vi "fp5.vi"   [LabVIEW 2016]
uses:
  <vilib>/NXT/Block Support/NXT_OutputPort.ctl
  <vilib>/NXT/Block Support/NXT_InputPort.ctl
  <vilib>/NXT/NXTIO Xnodes/NXTIONodeSubVIs/LEGOResetMotors.vi
  <vilib>/NXT/Dual Mode Library/Sensors/Touch_Released.vi
  <vilib>/NXT/Dual Mode Library/Sensors/EV3_Color_Reflect.vi
  <vilib>/NXT/NXTIO Xnodes/NXTIONodeSubVIs/NXTMoveMotors.vi
  <vilib>/NXT/NXTIO Xnodes/NXTIONodeSubVIs/NXTMotorRunDistance.vi
  <vilib>/NXT/NXTIO Xnodes/NXTIONodeSubVIs/NXTStopMotors.vi
  <vilib>/NXT/Dual Mode Library/Sound/PlayF.vi
  <vilib>/NXT/Dual Mode Library/Sound/PlayG.vi
  <vilib>/NXT/Subs/LVHSConnector.ctl
  <vilib>/NXT/NXTIO Xnodes/AddressXNode/NXTIOAddress.xnode
  <vilib>/NXT/NXTIO Xnodes/NXTIOXNode/NXTIO.xnode
  <vilib>/NXT/LegoClasses/BrickReference/BrickReference.lvclass
types:
  T1 = typedef "NXT_OutputPort.ctl" = u8
  T2 = typedef "NXT_InputPort.ctl" = u32
  T3 = typedef "LVHSConnector.ctl" = refnum<class "BrickReference.lvclass">
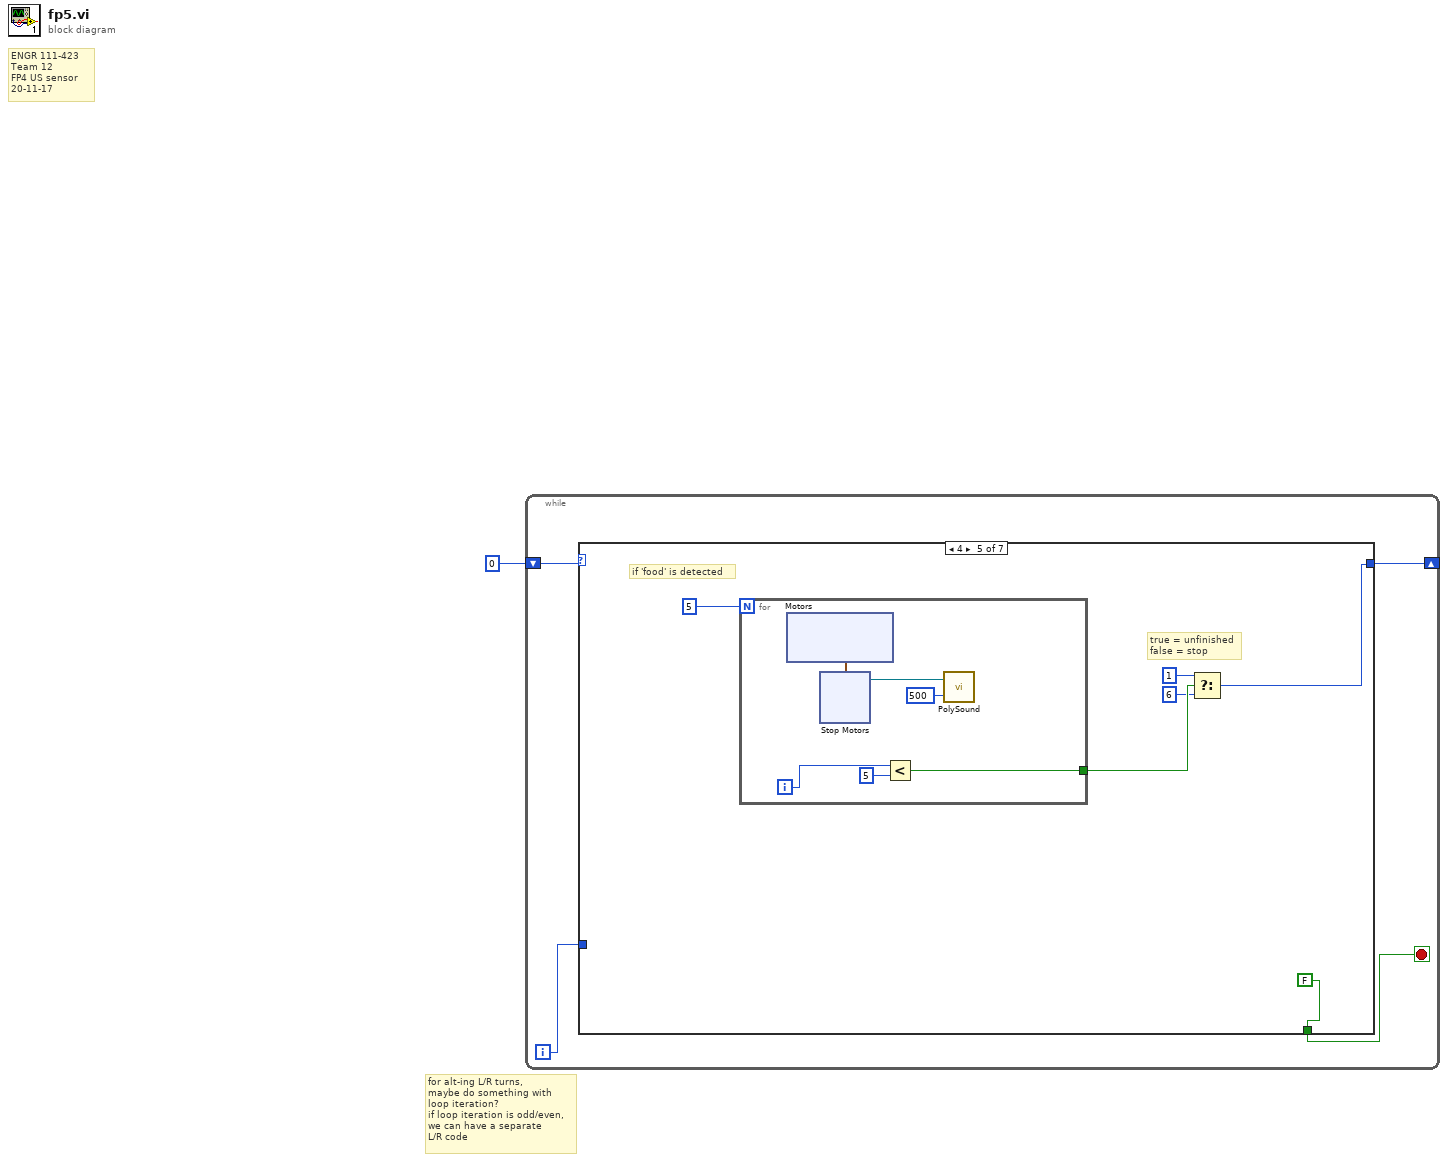
[diagram p0: block diagram]
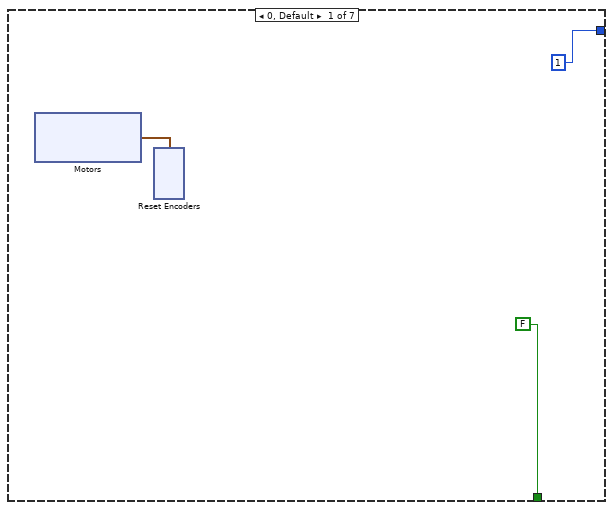
[diagram p2: hidden frame]
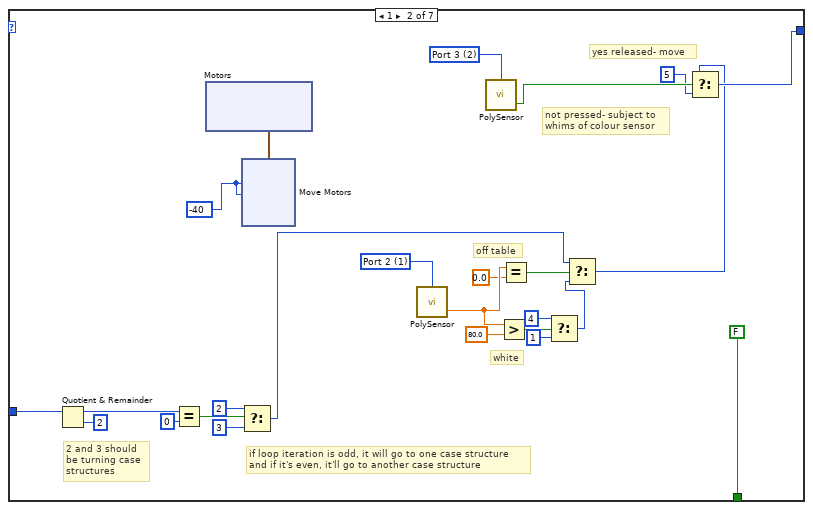
[diagram p3: hidden frame]
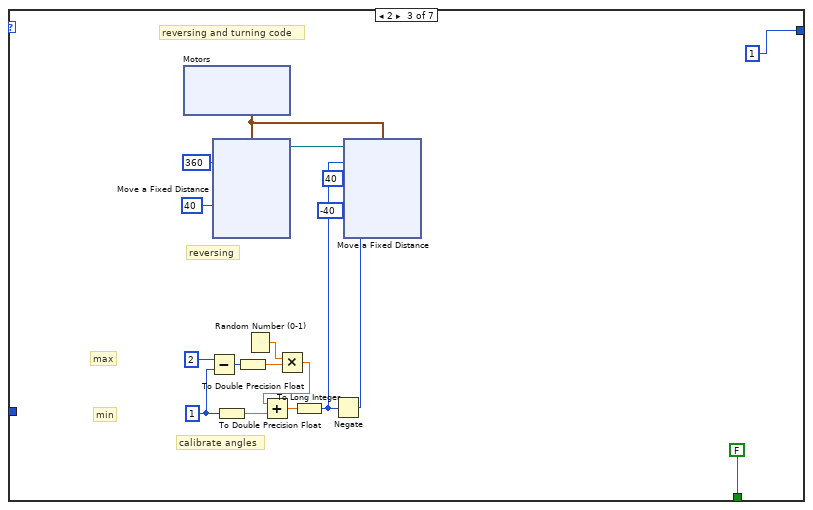
[diagram p4: hidden frame]
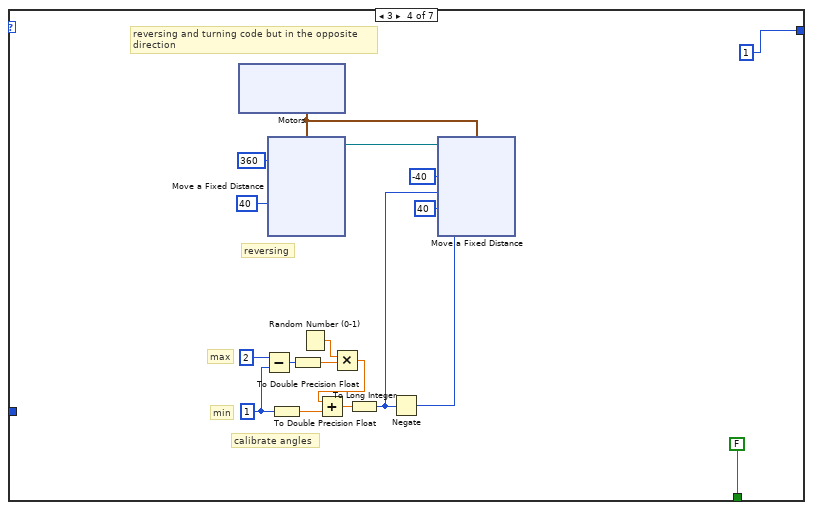
[diagram p5: hidden frame]
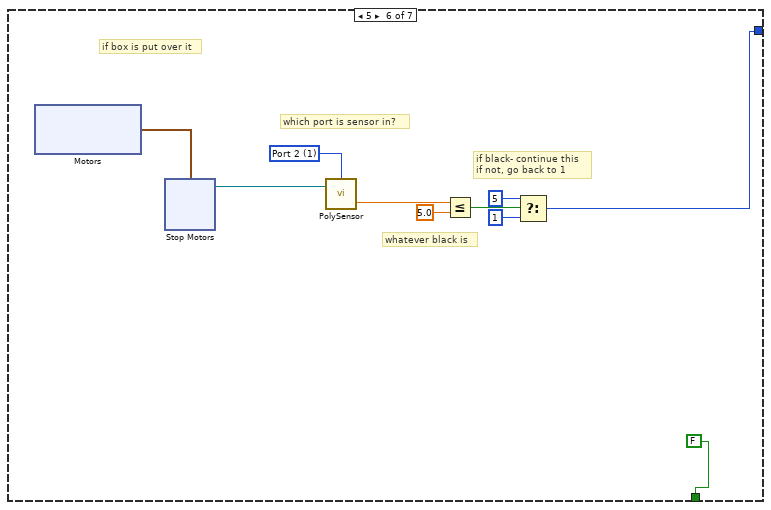
[diagram p6: hidden frame]
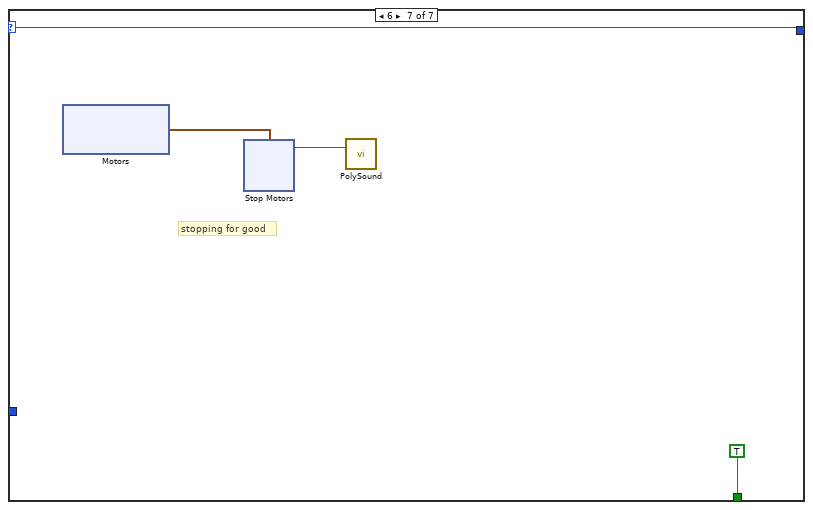
[diagram p7: hidden frame]
diagram:
  # "for alt-ing L/R turns,\nmaybe do something with\nloop iteration?\nif loop iteration is odd/even,\nwe can have a separate\nL/R code"
  # "ENGR 111-423\nTeam 12\nFP4 US sensor\n20-11-17"
  n1 = while {
    shift-right: [w3] -> _
    shift-left: 0 -> [w5]
    i -> [w2]
    stop <- w4 stop-if-true
    n2 = case shown="4" w5 {
      selector: w5 -> [_ _ _ _ _ _ w170]
      tunnel: [FALSE FALSE FALSE FALSE FALSE FALSE TRUE] -> w4
      tunnel: [1 w20 1 1 w135 w153 w170] -> w3
      tunnel: w2 -> [_ w33 _ _ _ _ _]
      frame 0, Default {
        n3 = xnode "Motors"() -> ("Motor"=w6:cluster{"Port":T1, "Port":T1})
        n4 = xnode "Reset Encoders"("Motors"=w6) -> ()  [unwired: 1 in, 1 out]
      }
      frame 1 {
        w21 = T2 1 items=["Port 1", "Port 2", "Port 3", "Port 4"] ("Port (Port 1)")
        w36 = T2 2 items=["Port 1", "Port 2", "Port 3", "Port 4"] ("Port (Port 1)")
        w37 = -40 ("Distance 1")
        # "white"
        # "off table"
        # "2 and 3 should\nbe turning case\nstructures"
        # "if loop iteration is odd, it will go to one case structure\nand if it's even, it'll go to another case structure"
        # "not pressed- subject to\nwhims of colour sensor"
        # "yes released- move"
        n5 = Quotient & Remainder(x=w33, y=2) -> (x-y*floor(x/y)=w31:i32)  [unwired: 1 out]
        n6 = Equal?(x=w31, y=0) -> (x = y?=w29:bool)
        n7 = xnode "Motors"() -> ("Motor"=w38:cluster{"Port":T1, "Port":T1})
        n8 = xnode "Move Motors"("Power/Speed 2"=w37, "Power/Speed 1"=w37, "Motors"=w38) -> ()  [unwired: 1 in, 1 out]
        n9 = Select(t=i16 2, s=w29, f=i16 3) -> (s? t:f=w18:i16)
        n10 = call-poly <vilib>:"PolySensor.vi"("Port (Port 1)"=w21) -> ("Scaled Value"=w22:sgl)  [unwired: 2 in, 1 out]
        n11 = call-poly <vilib>:"PolySensor.vi"("Port (Port 1)"=w36) -> ("Yes / No"=w35:bool)  [unwired: 2 in, 1 out]
        n12 = Greater?(x=w22, y=sgl 80.0) -> (0:w26:bool)
        n13 = Equal?(x=w22, y=sgl 0.0) -> (x = y?=w24:bool)
        n14 = Select(t=i16 4, s=w26, f=i16 1) -> (s? t:f=w17:i16)
        n15 = Select(t=w18, s=w24, f=w17) -> (s? t:f=w14:i16)
        n16 = Select(t=w14, s=w35, f=i16 5 ("t")) -> (s? t:f=w20:i16)
      }
      frame 2 {
        w58 = 1
        w64 = i8 40 ("Speed 2")
        w65 = 360 ("Distance 1")
        # "calibrate angles"
        # "min"
        # "max"
        # "reversing"
        # "reversing and turning code"
        n17 = xnode "Motors"() -> ("Motor"=w55:cluster{"Port":T1, "Port":T1})
        n18 = Subtract(x=2, y=w58) -> (x-y=w57:i32)
        n19 = xnode "Move a Fixed Distance"("Speed 2"=w64, "Speed 1"=w64, "Distance 2"=w65, "Distance 1"=w65, "Motors"=w55) -> ("NXT/EV3"=w54:T3)  [unwired: 1 in]
        n20 = To Double Precision Float(number=w58) -> (double precision float=w59:dbl)
        n21 = To Double Precision Float(number=w57) -> (double precision float=w60:dbl)
        n22 = Random Number (0-1)() -> (number: 0 to 1=w61:dbl)
        n23 = Multiply(x=w61, y=w60) -> (x*y=w63:dbl)
        n24 = Add(x=w63, y=w59) -> (x+y=w62:dbl)
        n25 = To Long Integer(number=w62) -> (32bit integer=w53:i32)
        n26 = Negate(x=w53) -> (-x=w52:i32)
        n27 = xnode "Move a Fixed Distance"("Speed 2"=i8 -40, "Speed 1"=i8 40, "Distance 2"=w52, "Distance 1"=w53, "Motors"=w55, "NXT/EV3"=w54) -> ()  [unwired: 1 out]
      }
      frame 3 {
        w104 = 1
        w98 = i8 40 ("Speed 2")
        w97 = 360 ("Distance 1")
        # "reversing and turning code but in the opposite\ndirection"
        # "calibrate angles"
        # "min"
        # "max"
        # "reversing"
        n28 = xnode "Motors"() -> ("Motor"=w107:cluster{"Port":T1, "Port":T1})
        n29 = Subtract(x=2, y=w104) -> (x-y=w105:i32)
        n30 = xnode "Move a Fixed Distance"("Speed 2"=w98, "Speed 1"=w98, "Distance 2"=w97, "Distance 1"=w97, "Motors"=w107) -> ("NXT/EV3"=w108:T3)  [unwired: 1 in]
        n31 = To Double Precision Float(number=w104) -> (double precision float=w103:dbl)
        n32 = To Double Precision Float(number=w105) -> (double precision float=w102:dbl)
        n33 = Random Number (0-1)() -> (number: 0 to 1=w101:dbl)
        n34 = Multiply(x=w101, y=w102) -> (x*y=w99:dbl)
        n35 = Add(x=w99, y=w103) -> (x+y=w100:dbl)
        n36 = To Long Integer(number=w100) -> (32bit integer=w94:i32)
        n37 = Negate(x=w94) -> (-x=w96:i32)
        n38 = xnode "Move a Fixed Distance"("Speed 2"=i8 40, "Speed 1"=i8 -40, "Distance 2"=w94, "Distance 1"=w96, "Motors"=w107, "NXT/EV3"=w108) -> ()  [unwired: 1 out]
      }
      frame 4 {
        # "true = unfinished\nfalse = stop"
        # "if 'food' is detected"
        n39 = for {
          N: 5 -> [_]
          tunnel: [w142] -> w138
          i -> [w144]
          n40 = xnode "Motors"() -> ("Motor"=w141:cluster{"Port":T1, "Port":T1})
          n41 = xnode "Stop Motors"("Motors"=w141) -> ("NXT/EV3"=w145:T3)  [unwired: 1 in]
          n42 = Less?(x=w144, y=5) -> (x < y?=w142:bool)
          n43 = call-poly <vilib>:"PolySound.vi"("Duration (500 ms)"=u16 500, "NXT/EV3"=w145) -> ()  [unwired: 2 in, 1 out]
        }
        n44 = Select(t=i16 1, s=w138, f=i16 6) -> (s? t:f=w135:i16)
      }
      frame 5 {
        w159 = T2 1 items=["Port 1", "Port 2", "Port 3", "Port 4"] ("Port (Port 1)")
        # "if black- continue this\nif not, go back to 1"
        # "whatever black is"
        # "which port is sensor in?"
        # "if box is put over it"
        n45 = xnode "Motors"() -> ("Motor"=w161:cluster{"Port":T1, "Port":T1})
        n46 = xnode "Stop Motors"("Motors"=w161) -> ("NXT/EV3"=w160:T3)  [unwired: 1 in]
        n47 = call-poly <vilib>:"PolySensor.vi"("NXT/EV3"=w160, "Port (Port 1)"=w159) -> ("Scaled Value"=w158:sgl)  [unwired: 1 in, 1 out]
        n48 = Less Or Equal?(x=w158, y=sgl 5.0) -> (x <= y?=w156:bool)
        n49 = Select(t=i16 5, s=w156, f=i16 1) -> (s? t:f=w153:i16)
      }
      frame 6 {
        # "stopping for good"
        n50 = xnode "Motors"() -> ("Motor"=w171:cluster{"Port":T1, "Port":T1})
        n51 = xnode "Stop Motors"("Motors"=w171) -> ("NXT/EV3"=w168:T3)  [unwired: 1 in]
        n52 = call-poly <vilib>:"PolySound.vi"("NXT/EV3"=w168) -> ()  [unwired: 3 in, 1 out]
      }
    }
  }
